vi "Codec Selector (SubVi).vi"(8 "error in (no error)":errorcluster, 11 "Array":string[](array[string])) -> (0 "error out":errorcluster, 3 "String":string)   [LabVIEW 2023]
panel:
  in  "Continue":bool
  in  "Codec Selector":u16(ring) items=["Test", "Retext"]
  # "The selected codec is not in the list of available codecs\nor you have opted to select at runtime\nPlease select the desired codec"
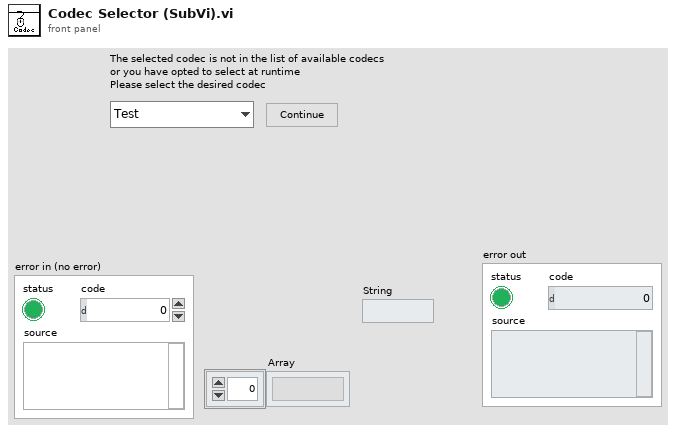
[diagram p1: front panel]
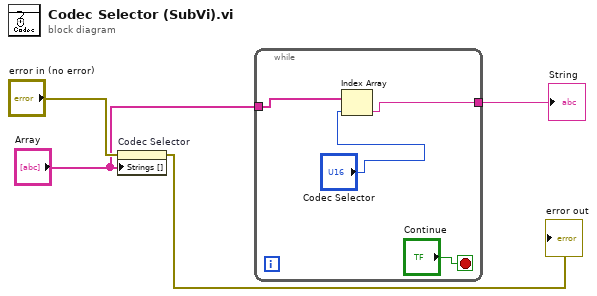
[diagram p0: block diagram]
diagram:
  n1 = property on="Codec Selector" class="Ring (strict)"(error in="error in (no error)", "Strings []"="Array") -> (error out=→"error out":errorcluster)  [unwired: 1 in, 1 out]
  n2 = while {
    tunnel: "Array" -> [w7]
    tunnel: [w5] -> w1
    stop <- "Continue" stop-if-true
    n3 = Index Array(array=w7, index="Codec Selector") -> (element=w5:string)
  }
  "String" <- w1
